vi "hasElement.vi"(8 "error in (no error)":errorcluster, 10 "Name":string, 11 "tBSONDocument in":refnum<class "tBSONDocument.lvclass">) -> (0 "error out":errorcluster, 2 "hasElement":bool, 3 "tBSONDocument out":refnum<class "tBSONDocument.lvclass">)   [LabVIEW 2013, in "BSON.lvlib" / "tBSONDocument.lvclass"]
doc: "Checks the document to see if an element with the name specified exists."
uses:
  tBSONDocument.lvclass
  tBSONDocument.lvclass/tBSONDocument.ctl
  BSONElements/tBSONDocumentElement/tBSONDocumentElement.lvclass
  BSONElements/tBSONDocumentElement/getValue.vi
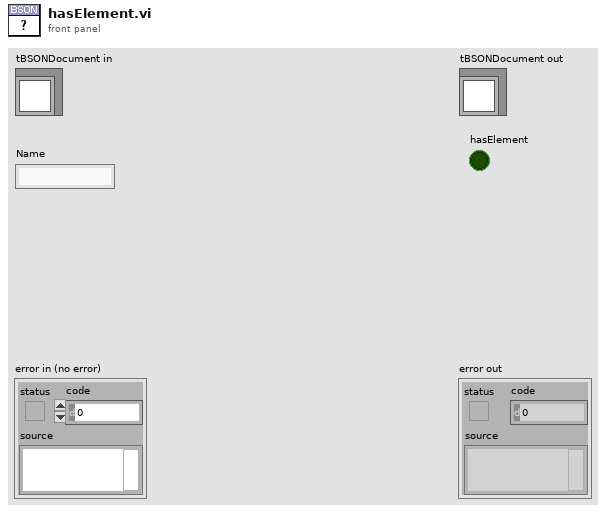
[diagram p1: front panel]
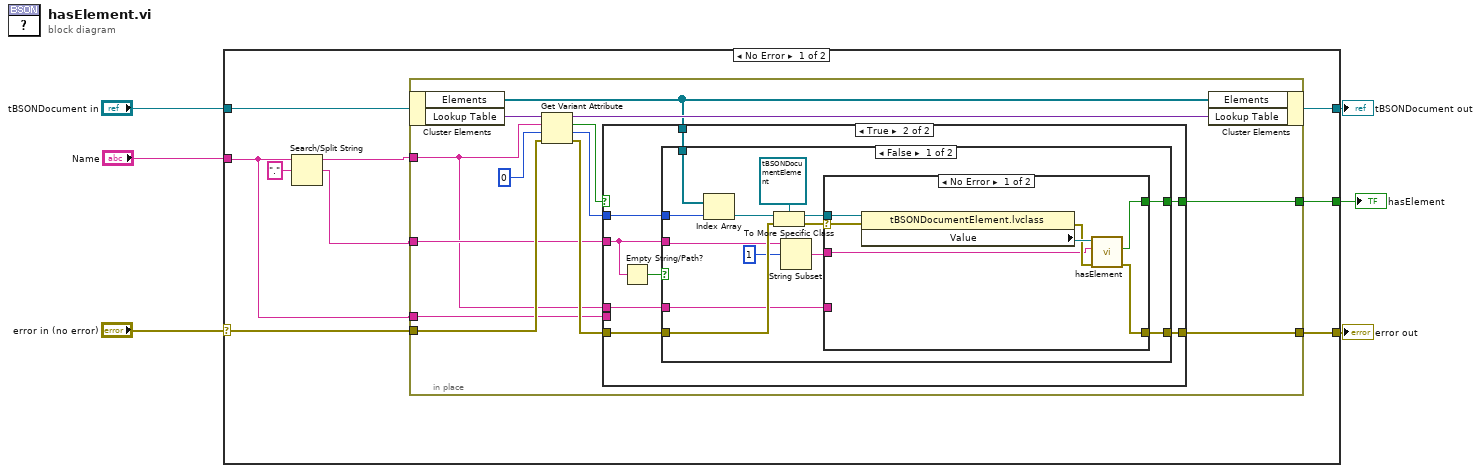
[diagram p0: block diagram]
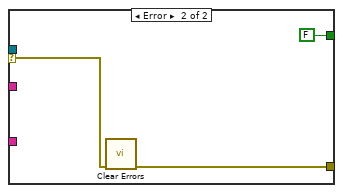
[diagram p3: hidden frame]
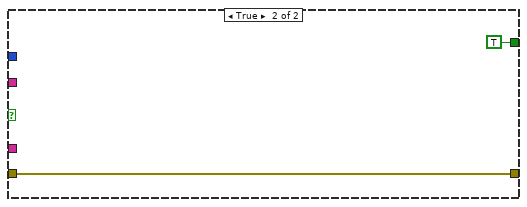
[diagram p4: hidden frame]
diagram:
  n1 = case shown="No Error" "error in (no error)" {
    selector: "error in (no error)" -> [w9 w65]
    tunnel: [w8 w65] -> w5
    tunnel: "tBSONDocument in" -> [w15 w64]
    tunnel: "Name" -> [w10 _]
    tunnel: [w14 w64] -> w2
    tunnel: [w7 _] -> w1
    frame No Error {
      n2 = Search/Split String(string=w10, search string/char (-)=".") -> (substring before match=w12:string, match + rest of string=w11:string)  [unwired: 1 in, 1 out]
      n3 = in-place {
        in-place-border: w9 -> [w27]
        in-place-border: w12 -> [w18]
        in-place-border: w11 -> [w21]
        in-place-border: [w20] -> w8
        in-place-border: w10 -> [w19]
        in-place-border: [w17] -> w7
        n4 = in-place-cluster #1(w15) -> ("Elements"=w16:refnum<class "tBSONElement.lvclass">[], "Lookup Table"=w28:variant)
        n5 = Get Variant Attribute(Variant=w28, name=w18, default value (empty Variant)=0, error in=w27) -> (duplicate Variant=w25:variant, found=w24:bool, value=w22:i32, error out=w23:errorcluster)
        n6 = case shown="True" w24 {
          selector: w24 -> [w29 _]
          tunnel: w23 -> [w30 w37]
          tunnel: w22 -> [_ w31]
          tunnel: w21 -> [_ w35]
          tunnel: [w30 w36] -> w20
          tunnel: w19 -> [_ _]
          tunnel: w18 -> [_ w34]
          tunnel: [w29 w33] -> w17
          tunnel: w16 -> [_ w32]
          frame False {
          }
          frame True {
            n7 = Empty String/Path?(string/path=w35) -> (empty?=w38:bool)
            n8 = case shown="False" w38 {
              tunnel: w37 -> [w50 w63]
              tunnel: [w47 w63] -> w36
              tunnel: w35 -> [w45 _]
              tunnel: w34 -> [w46 _]
              tunnel: [w42 TRUE ("Has Name?")] -> w33
              tunnel: w32 -> [w41 _]
              tunnel: w31 -> [w40 _]
              frame False {
                n9 = Index Array(array=w41, index=w40) -> (element=w39:refnum<class "tBSONElement.lvclass">)
                n10 = To More Specific Class(target class=refnum<class "tBSONDocumentElement.lvclass"> refnum ("BSON.lvlib:tBSONDocumentElement.lvclass"), reference=w39, error in=w50) -> (specific class reference=w48:refnum<class "tBSONDocumentElement.lvclass">, error out=w49:errorcluster)
                n11 = String Subset(string=w45, offset (0)=1) -> (substring=w43:string)  [unwired: 1 in]
                n12 = case shown="No Error" w49 {
                  selector: w49 -> [w58 w60]
                  tunnel: w48 -> [w57 _]
                  tunnel: w43 -> [w54 _]
                  tunnel: [w52 w59] -> w47
                  tunnel: w46 -> [_ _]
                  tunnel: [w53 FALSE] -> w42
                  frame No Error {
                    n13 = property class="tBSONDocumentElement.lvclass"(reference=w57, error in=w58) -> (error out=w55:errorcluster, "Value"=w56:refnum<class "tBSONDocument.lvclass">)  [unwired: 1 out]
                    n14 = call "hasElement.vi"("error in (no error)"=w55, "Name"=w54, "tBSONDocument in"=w56) -> ("error out"=w52:errorcluster, "hasElement"=w53:bool)  [unwired: 6 in, 1 out]
                  }
                  frame Error {
                    n15 = call <vilib>:"Clear Errors.vi"("error in (no error)"=w60) -> ("error out"=w59:errorcluster)  [unwired: 6 in]
                  }
                }
              }
              frame True {
              }
            }
          }
        }
        n16 = in-place-cluster #1("Elements"=w16, "Lookup Table"=w25) -> (w14:refnum<class "tBSONDocument.lvclass">)
      }
    }
    frame Error {
    }
  }
  "error out" <- w5
  "tBSONDocument out" <- w2
  "hasElement" <- w1
